vi "Acknowledge Faults.vi"(0 "object in":refnum<class "HPS-17000-PowerModule.lvclass">, 11 "Error In":errorcluster) -> (4 "object out":refnum<class "HPS-17000-PowerModule.lvclass">, 15 "Error Out":errorcluster)   [LabVIEW 2023, in "HPS-17000-PowerModule.lvlib" / "HPS-17000-PowerModule.lvclass"]
uses:
  HPS-17000-PowerModule.lvclass
  <instrlib>/HPS-17000/Internal/Acknowledge Faults Multi.vi
  <instrlib>/HPS-17000/HPS-17000.lvclass
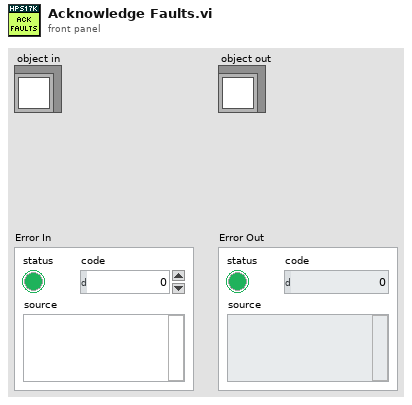
[diagram p1: front panel]
types:
  T1 = typedef "HPS-17000-PowerModule.lvlib/HPS-17000-PowerModule.lvclass/ObjectAttributes.ctl" = cluster{"JSON Config Path":path, "Configuration":T2, "GM ID":string, "HPS17000 Refs":refnum<class "HPS-17000.lvclass">[], "connected":bool, "reserved":bool, "events":T4, "nibatterycycler_grpc_Setpoint":T5, "last timestamp":i64, "mode":T6, "range":T7, "measurement array":T8[], "measurement stream":bool, "setpoint stream":bool}
  T2 = typedef "HPS-17000-PowerModule.lvlib/HPS-17000-PowerModule.lvclass/Configuration.ctl" = cluster{"TSN NIC IP Address":string, "HPS17000 IP Addresses":string[], "HPS Topology":enum16{"SINGLE", "MULTI"}, "Setpoint Stream Config":T3, "Measurement Array Size":i32}
  T3 = typedef "Cycler.lvclass/Setpoint Stream Basic Config.ctl" = cluster{"local address":string, "receiver port":u16}
  T4 = typedef "HPS-17000.lvclass/Multi-Cycler Events.ctl" = cluster{"heartbeats events":refnum<user-event>[], "faults events":refnum<user-event>[], "network sync event":refnum<user-event>[], "setpoint status event":refnum<user-event>[]}
  T5 = typedef "NI_BC_client.lvlib/nibatterycycler_grpc_Setpoint.ctl" = cluster{"voltage":sgl, "current":sgl, "min_power":sgl, "max_power":sgl, "resistance":sgl}
  T6 = typedef "HPS-17000-PowerModule.lvlib/HPS-17000-PowerModule.lvclass/Mode.ctl" = u16
  T7 = typedef "PowerModuleInterface.lvlibp/PowerModuleInterface.lvclass/Range.ctl" = cluster{"Current Max (A)":dbl, "Current Min (A)":dbl, "Voltage Max (V)":dbl, "Voltage Min (V)":dbl}
  T8 = typedef "PowerModuleInterface.lvlibp/PowerModuleInterface.lvclass/Measurements.ctl" = cluster{"measured voltage (V)":dbl, "measured current (A)":dbl, "setpoint voltage (V)":dbl, "setpoint current (A)":dbl, "timestamp":dbl}
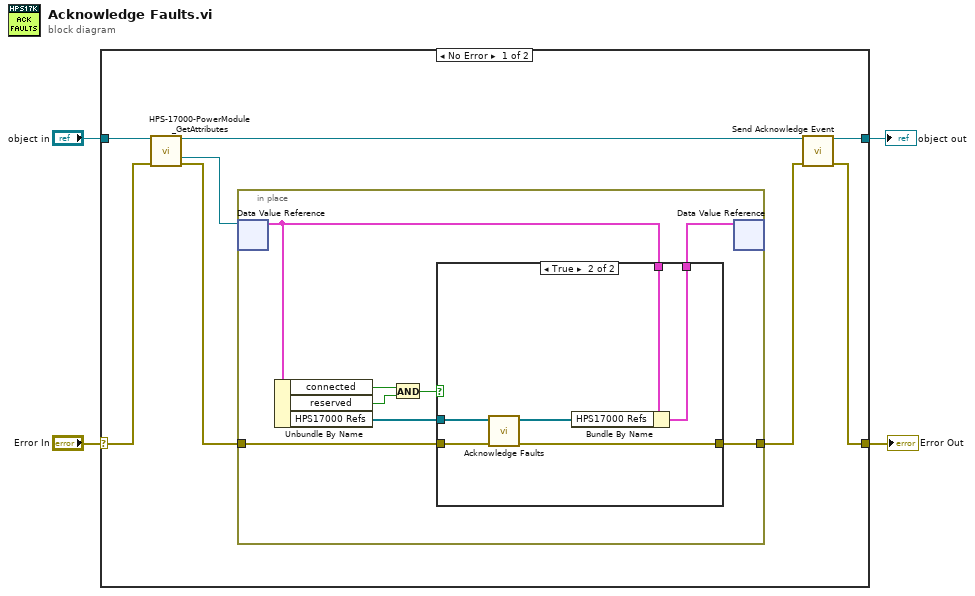
[diagram p0: block diagram]
diagram:
  n1 = case shown="No Error" "Error In" {
    selector: "Error In" -> [w11 w29]
    tunnel: "object in" -> [w12 w30]
    tunnel: [w6 w30] -> w4
    tunnel: [w5 w29] -> w2
    frame No Error {
      n2 = call "HPS-17000-PowerModule_GetAttributes.vi"("reference in"=w12, "Error In"=w11) -> ("reference out"=w7:refnum<class "HPS-17000-PowerModule.lvclass">, "DataRef"=w10:refnum<data-value>, "Error Out"=w9:errorcluster)  [unwired: 10 in, 1 out]
      n3 = in-place {
        in-place-border: w9 -> [w18]
        in-place-border: [w17] -> w8
        n4 = in-place-dvr #1(w10) -> (w19:T1)  [unwired: 1 out]
        n5 = Unbundle By Name(w19) -> ("connected"=w15:bool, "reserved"=w14:bool, "HPS17000 Refs"=w16:refnum<class "HPS-17000.lvclass">[])
        n6 = And(x=w15, y=w14) -> (x .and. y?=w13:bool)
        n7 = case shown="True" w13 {
          tunnel: [w22 w28] -> w20
          tunnel: w19 -> [w22 w27]
          tunnel: w18 -> [w21 w25]
          tunnel: [w21 w24] -> w17
          tunnel: w16 -> [_ w26]
          frame False {
          }
          frame True {
            n8 = call-poly <instrlib>:"Acknowledge Faults.vi"("error in"=w25, "cycler refs in"=w26) -> ("error out"=w24:errorcluster, "cycler refs out"=w23:refnum<class "HPS-17000.lvclass">[])  [unwired: 8 in]
            n9 = Bundle By Name(cluster=w27, "HPS17000 Refs"=w23) -> (w28:T1)
          }
        }
        n10 = in-place-dvr #1(w20) -> ()  [unwired: 2 out]
      }
      n11 = call "Send Acknowledge Event.vi"("reference in"=w7, "Error In"=w8) -> ("reference out"=w6:refnum<class "HPS-17000-PowerModule.lvclass">, "Error Out"=w5:errorcluster)  [unwired: 12 in]
    }
    frame Error {
    }
  }
  "Error Out" <- w2
  "object out" <- w4
